vi "2023_day10(SubVI Table Element BG Color).vi"(7 "Table in":refnum<vi>, 8 "Color (White)":u32(colorbox)=16448250, 10 "Position":i32[](array[numeric])) -> ()   [LabVIEW 2021]
uses:
  <vilib>/Utility/miscctls.llb/LVRowAndColumnTypeDef.ctl
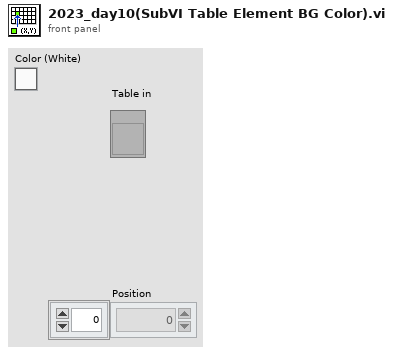
[diagram p1: front panel]
types:
  T1 = typedef "LVRowAndColumnTypeDef.ctl" = cluster{"Row":i32, "Column":i32}
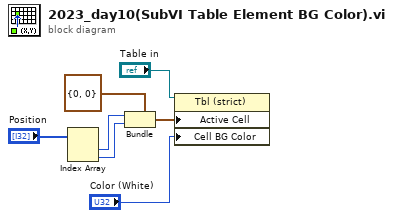
[diagram p0: block diagram]
diagram:
  n1 = Index Array(array="Position") -> (element #1=w5:i32, element #2=w6:i32)  [unwired: 2 in]
  n2 = Bundle(cluster=T1 {"Row"=0, "Column"=0} ("Active Cell:Active Cell"), "Row"=w5, "Column"=w6) -> (w2:T1)
  n3 = property on="Property Node" class="Tbl (strict)"(reference="Table in", "Active Cell"=w2, "Cell BG Color"="Color (White)") -> ()  [unwired: 1 in, 2 out]
